vi "ResistanceInputStart.vi"(0 "Device Info":T1={"Serial Number"=-1, "Channel"=0, "Port"=0}, 1 "Data Interval":i32=-1, 2 "Change Trigger":dbl, 5 "RTD Wire Setup":u32(ring)=3 items=["RTD_WIRE_SETUP_2WIRE"=1, "RTD_WIRE_SETUP_3WIRE"=2, "RTD_WIRE_SETUP_4WIRE"=3], 11 "error in (no error)":errorcluster, 12 "Connection":u16(ring) items=["No Preference", "Remote", "Local"], 13 "Timeout (mSec)":i32=5000) -> (4 "Phidget ID":u64, 6 "Serial Number Return":i32, 10 "Attached?":bool, 15 "error out":errorcluster)   [LabVIEW 2020, in "Phidget Resistance Input.lvlib"]
doc: "${ResistanceInput:StartHeader}"
uses:
  <instrlib>/Phidgets/Phidget Resistance Input/Phidget Resistance Input.lvlib
  <instrlib>/Phidgets/Phidget Common/Phidget Common.lvlib
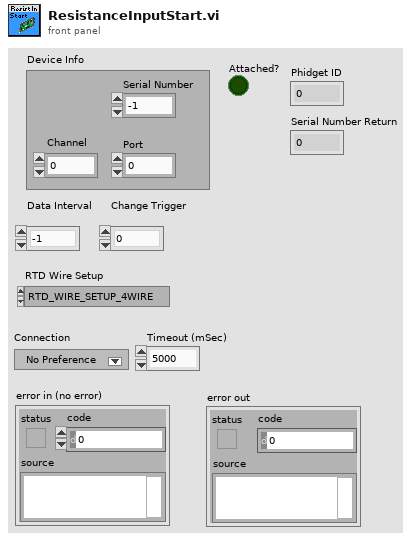
[diagram p1: front panel]
types:
  T1 = cluster{"Serial Number":i32, "Channel":i32, "Port":i32}
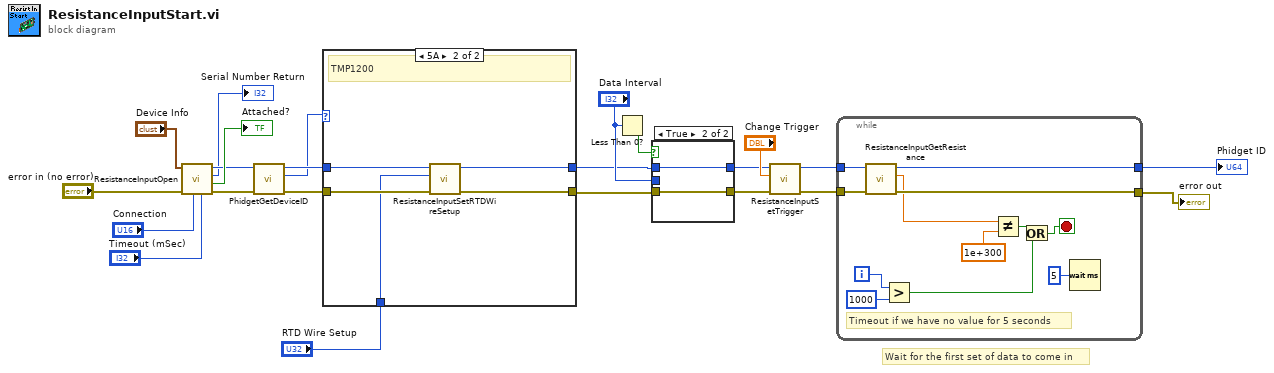
[diagram p0: block diagram]
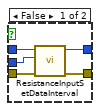
[diagram p2: hidden frame]
diagram:
  # "Wait for the first set of data to come in"
  n1 = call <instrlib>:"ResistanceInputOpen.vi"("Timeout (mSec)"="Timeout (mSec)", "Connection"="Connection", "error in"="error in (no error)", "Device Info"="Device Info") -> ("error out"=w20:errorcluster, "Attached?"=→"Attached?":bool, "Serial Number Return"=→"Serial Number Return":i32, "Phidget ID"=w19:u64)  [unwired: 4 in]
  n2 = call <instrlib>:"PhidgetGetDeviceID.vi"("error in (no error)"=w20, "Device In"=w19) -> ("error out"=w13:errorcluster, "Devie IDs"=w12:u32, "Device Out"=w14:u64)  [unwired: 6 in]
  n3 = case shown="5A" w12 {
    tunnel: w14 -> [w25 w30]
    tunnel: w13 -> [w24 w29]
    tunnel: [w25 w27] -> w4
    tunnel: [w24 w26] -> w2
    tunnel: "RTD Wire Setup" -> [_ w28]
    frame 0, Default {
    }
    frame 90 {
      # "TMP1200"
      n4 = call <instrlib>:"ResistanceInputSetRTDWireSetup.vi"("error in (no error)"=w29, "RTD Wire Setup"=w28, "Device In"=w30) -> ("error out"=w26:errorcluster, "Device Out"=w27:u64)  [unwired: 6 in]
    }
  }
  n5 = Less Than 0?(x="Data Interval") -> (x < 0?=w6:bool)
  n6 = case shown="True" w6 {
    tunnel: w4 -> [w34 w37]
    tunnel: w2 -> [w35 w36]
    tunnel: [w33 w37] -> w3
    tunnel: [w32 w36] -> w1
    tunnel: "Data Interval" -> [w31 _]
    frame False {
      n7 = call <instrlib>:"ResistanceInputSetDataInterval.vi"("error in (no error)"=w35, "Interval"=w31, "Device In"=w34) -> ("error out"=w32:errorcluster, "Device Out"=w33:u64)  [unwired: 6 in]
    }
    frame True {
    }
  }
  n8 = call <instrlib>:"ResistanceInputSetTrigger.vi"("error in (no error)"=w1, "Trigger"="Change Trigger", "Device In"=w3) -> ("error out"=w15:errorcluster, "Device Out"=w16:u64)  [unwired: 6 in]
  n9 = while {
    tunnel: w16 -> [w47]
    tunnel: w15 -> [w46]
    tunnel: [w44] -> w18
    tunnel: [w45] -> w22
    i -> [w39]
    stop <- w41 stop-if-true
    # "Timeout if we have no value for 5 seconds"
    n10 = call <instrlib>:"ResistanceInputGetResistance.vi"("error in (no error)"=w46, "Device In"=w47) -> ("error out"=w45:errorcluster, "Resistance"=w38:dbl, "Device Out"=w44:u64)  [unwired: 6 in]
    n11 = Greater?(x=w39, y=1000) -> (0:w42:bool)
    n12 = Not Equal?(x=w38, y=1e+300) -> (x != y?=w43:bool)
    n13 = Or(x=w43, y=w42) -> (x .or. y?=w41:bool)
    n14 = Wait (ms)(milliseconds to wait=u32 5) -> ()  [unwired: 1 out]
  }
  "error out" <- w22
  "Phidget ID" <- w18
